vi "JLINK EraseChip.vi"(8 "error in (no error)":errorcluster) -> (0 "error out":errorcluster, 3 "Return value":i32)   [LabVIEW 2020, in "JLinkARM.lvlib"]
uses:
  Lib/JLinkARM.lvlib
  JLinkARM.dll
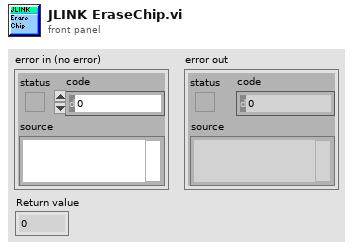
[diagram p1: front panel]
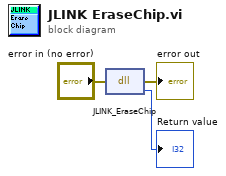
[diagram p0: block diagram]
diagram:
  n1 = dll-call lib="C:/Users/anybody/Desktop/JLinkARM.dll" fn="JLINK_EraseChip"(error in="error in (no error)") -> (error out=→"error out":errorcluster, "return type"=→"Return value":i32)  [unwired: 2 in, 1 out]
